vi "Num to Bool Array.vi"(9 "Array Size":i32, 11 "Value":u8) -> (3 "Bool Array":bool[](array[boolean]))   [LabVIEW 2017, in "2D Plot.lvclass"]
uses:
  <vilib>/Math Plots/2D Math Plots/2D Plot/2D Plot/2D Plot.lvclass
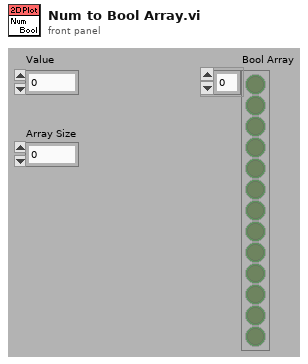
[diagram p1: front panel]
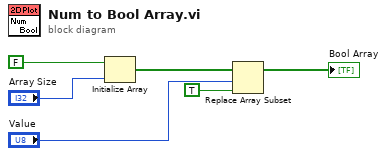
[diagram p0: block diagram]
diagram:
  n1 = Initialize Array(FALSE, "Array Size") -> (w4:bool[])
  n2 = Replace Array Subset(array=w4, new element=TRUE, index="Value") -> (→"Bool Array":bool[])
